vi "Read Write ASCII-Unicode Text File modified.vi"(2 "String Out":string, 8 "error in":errorcluster) -> (0 "error out":errorcluster, 3 "file path Out":path)   [LabVIEW 2011]
uses:
  Sub VIs/Unicode files/File IO/Read Write AU Text File option.ctl
  Sub VIs/Unicode files/File IO/Text Encoding Format.ctl
panel:
  in  "Boolean":bool
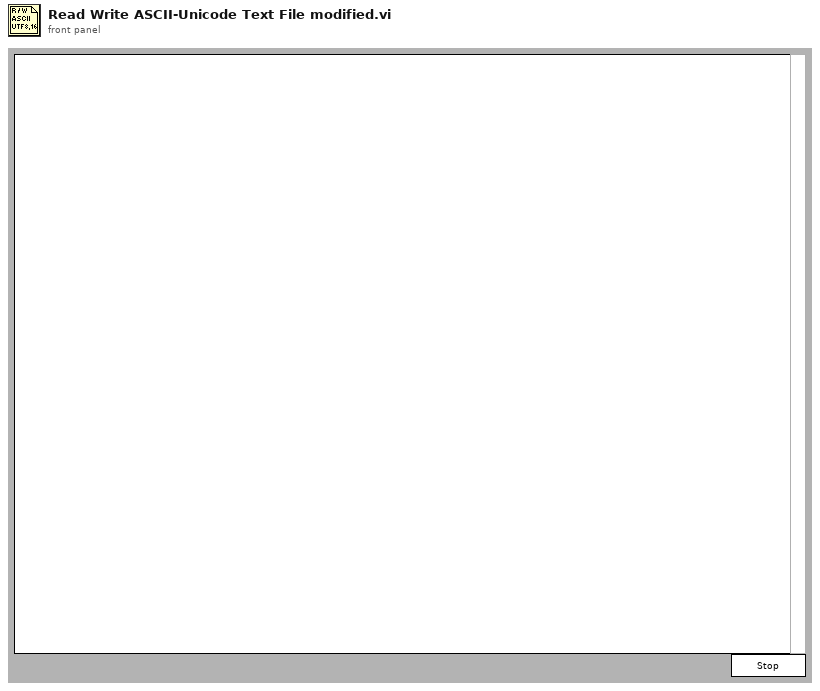
[diagram p1: front panel]
types:
  T1 = typedef "Text Encoding Format.ctl" = enum8{"ASCII", "UTF-8", "UTF-16 LE", "UTF-16 BE"}
  T2 = typedef "Read Write AU Text File option.ctl" = enum16{"Read", "Write"}
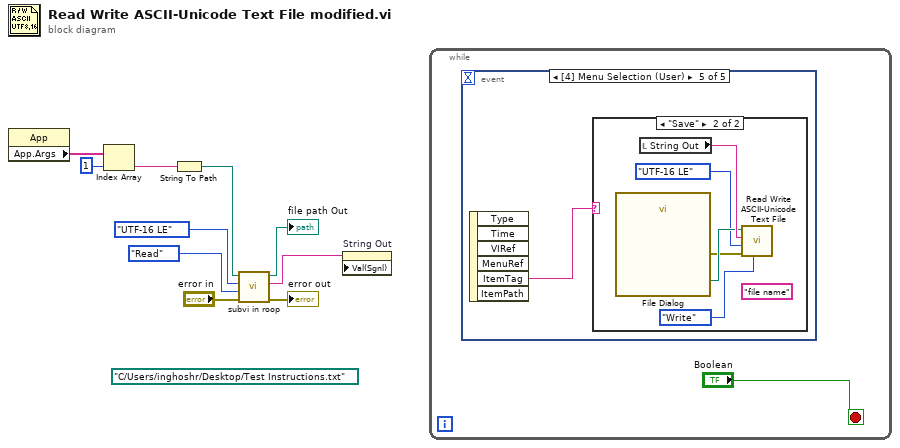
[diagram p0: block diagram]
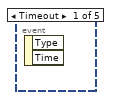
[diagram p2: hidden frame]
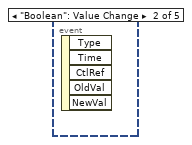
[diagram p3: hidden frame]
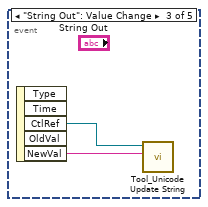
[diagram p4: hidden frame]
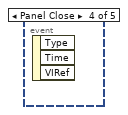
[diagram p5: hidden frame]
diagram:
  (unwired) path "C:/Users/inghoshr/Desktop/Test Instructions.txt"
  n1 = property class="App"() -> ("App.Args"=w7:string[])  [unwired: 2 in, 2 out]
  n2 = Index Array(array=w7, index=1) -> (element=w5:string)
  n3 = String To Path(string=w5) -> (path=w1:path)
  n4 = call "subvi in roop.vi"("error in"="error in", "Option"=Read_Write_AU_Text_File_option."Read", "Encoding?"=Text_Encoding_Format."UTF-16 LE", "Path in"=w1) -> ("error out"=→"error out":errorcluster, "UTF-8 String"=w2:string, "Path out"=→"file path Out":path)  [unwired: 5 in]
  n5 = property on="String Out" class="Str"("Val(Sgnl)"=w2) -> ()  [unwired: 2 in, 2 out]
  n6 = while {
    stop <- "Boolean" stop-if-true
    n7 = event shown="[4] Menu Selection (User)" {
      selector: _ -> [_ _ _ _ _]
      dyn-events: _ -> [_ _ _ _ _]
      timeout: _ -> [_ _ _ _ _]
      event Timeout {
        n8 = event-data() -> ()  [unwired: 1 in, 2 out]
      }
      event "Boolean": Value Change {
        n9 = event-data() -> ()  [unwired: 1 in, 5 out]
      }
      event "String Out": Value Change {
        n10 = event-data() -> ("CtlRef"=w12:refnum<vi>, "NewVal"=w13:string)  [unwired: 1 in, 3 out]
        n11 = call "Tool_Unicode Update String.vi"("String Value"=w13, "String Control Reference"=w12) -> ()  [unwired: 6 in, 2 out]
      }
      event Panel Close {
        n12 = event-data() -> ()  [unwired: 1 in, 3 out]
      }
      event Menu Selection (User) {
        n13 = event-data() -> ("ItemTag"=w14:string)  [unwired: 1 in, 5 out]
        n14 = case shown="\"Save\"" w14 {
          frame "False", Default {
          }
          frame "Save" {
            (unwired) "file name" ("prompt (Choose or enter file path)")
            n15 = call "File Dialog"() -> ("selected path"=w18:path, "error out"=w17:errorcluster)  [unwired: 12 in, 2 out]
            n16 = local read "String Out"() -> (w19:string)
            n17 = call "Read Write ASCII-Unicode Text File.vi"("Option"=Read_Write_AU_Text_File_option."Write", "error in"=w17, "Encoding?"=Text_Encoding_Format."UTF-16 LE", "String In"=w19, "file path"=w18) -> ()  [unwired: 4 in, 3 out]
          }
        }
      }
    }
  }
